vi "FPGA Main.vi"() -> ()   [LabVIEW 2013]
doc: "This FPGA Main VI contains a control loop running in parallel with an RT watchdog loop.\n- The Control Loop performs control calculations on four input channels in parallel, and outputs the results to four output channels.\n- The RT Watchdog Loop checks for a periodic 'pet' from the RT Main VI to ensure communications between RT and FPGA are maintained."
uses:
  controls/FPGA State.ctl
  controls/Control Configuration.ctl
  controls/Raw Values.ctl
  <vilib>/LabVIEW Targets/FPGA/cRIO/cRIO-9505/controls.llb/_nicrio_cRIO-9505_DriveStatus.ctl
  controls/Custom Controller Inputs.ctl
  controls/Controller Calcs.ctl
  controls/Observer Calcs.ctl
  controls/Other Calcs.ctl
  <vilib>/Platform/TimedLoop/XDataNode/timing_clust.ctl
  <vilib>/Platform/TimedLoop/XDataNode/nitl_modes.ctl
  <vilib>/Platform/TimedLoop/XDataNode/wakeup.ctl
  <vilib>/LabVIEW Targets/FPGA/cRIO/cRIO-9505/controls.llb/_nicrio_cRIO-9505_DriveDirection.ctl
  <vilib>/rvi/Emulation/niFpgaSctlEmulationGetInTimedLoop.vi
  <vilib>/rvi/Emulation/niFpgaEmulationReportErrorSimple.vi
  <vilib>/rvi/Emulation/niFpgaGetClockAttributes.vi
  <vilib>/rvi/Emulation/niFpgaCriticalErrorInLSC.vi
  <vilib>/rvi/Emulation/niFpgaProcessEmulError.vi
  <vilib>/rvi/eio/common/nirviEmuTemplateMethod_errors.vi
  <vilib>/rvi/eio/common/nirviEmuTemplatePropertyGet_noerrors.vi
  <vilib>/Platform/TimedLoop/XDataNode/XDataNode.xnode
  <vilib>/eio/EIONode/EIONode.xnode
  <vilib>/eio/EIOMethodNode/EIOMethodNode.xnode
  <vilib>/eio/EIOPropertyNode/EIOPropertyNode.xnode
  <vilib>/rvi/Analysis/measure/butterworth/XNode/niFpgaButterworthFilter.xnode
  <vilib>/Platform/TimedLoop/XDataNode/XDNodeRunTimeDep.lvlib
  <vilib>/rvi/eio/common/nirviEmuTemplatePropertyGet_errors.vi
  <vilib>/rvi/eio/common/nirviEmuTemplatePropertySet_errors.vi
  <vilib>/rvi/eio/common/nirviEmuTemplatePropertySet_noerrors.vi
panel:
  out "Other Calcs":T1
  out "Observer Calcs":T2
  out "Controller Calcs":T3
  in  "Reset Integrator":bool
  in  "Custom Controller Inputs":T4={"Other Controller Gains"={"kvc (N/m)"=3000.0, "ymod (-)"=0.0, "Mar (kg)"=0.0, "bp (kg/s)"=0.0, "Foff (N)"=0.0, "Fthresh (N)"=2.0}}
  in  "Mod1/AO4":fxp<+,16,3>
  in  "Trig AI":bool
  out "Vsup Present":bool
  out "Drive Fault":bool
  out "Drive Status":T5=enum."Disabled"
  out "Temp Fault":bool
  in  "Enable\nDrive":bool
  in  "Disable\nDrive":bool
  out "PWM Duty Cycle":i16
  out "F_Error (N)":fxp<+/-,40,11>
  in  "Force Sensor Gain (N/V)":fxp<+,20,6>=53.02703857421875
  in  "L12 Offset (mA)":fxp<+,18,4>=1.0
  in  "L12 Gain (mA/N)":fxp<+,16,2>=1.0
  out "Measured Force (N)":fxp<+,39,10>
  out "Controller\nOutput":fxp<+,18,3>
  in  "Channel 3 Setpoint":fxp<+/-,16,7>
  in  "Channel 2 Setpoint":fxp<+/-,20,7>
  in  "Channel 1 Setpoint  (Position)":fxp<+/-,20,7>=25.0
  in  "Channel 0 Setpoint (Force)":fxp<+/-,20,7>
  out "Watchdog Timed Out?":bool=TRUE
  in  "Enable Watchdog":bool
  in  "Pet Watchdog":bool
  in  "Watchdog Timeout Period (ticks)":u64=40000000 format="%.0p"
  out "Time Since Last Pet":u64
  in  "Manual Values":T6
  out "Output Values":T6
  out "Input Values":T6
  in  "Channel 3 Configuration":T7={"PID Gains"={"proportional gain (Kc)"=0.0, "integral gain (Kc*Ts/Ti)"=0.0, "derivative gain (Kc*Td/Ts)"=0.0}, "Output Range"={"output high"=10.0, "output low"=-10.0}}
  in  "Channel 2 Configuration":T7={"PID Gains"={"proportional gain (Kc)"=0.0, "integral gain (Kc*Ts/Ti)"=0.0, "derivative gain (Kc*Td/Ts)"=0.0}, "Output Range"={"output high"=10.0, "output low"=-10.0}}
  in  "Channel 1 Configuration":T7={"PID Gains"={"proportional gain (Kc)"=0.0, "integral gain (Kc*Ts/Ti)"=0.0, "derivative gain (Kc*Td/Ts)"=0.0}, "Output Range"={"output high"=10.0, "output low"=-10.0}}
  in  "Channel 0 Configuration":T7={"PID Gains"={"proportional gain (Kc)"=55.0, "integral gain (Kc*Ts/Ti)"=0.0, "derivative gain (Kc*Td/Ts)"=0.0}, "Output Range"={"output high"=50.0, "output low"=-50.0}}
  in  "New State":T8=enum."Control (PID)"
  out "Actual Loop Period (ticks)":u32
  out "Current FPGA State":T8=enum."Manual"
  in  "Change State":bool
  out "Input Error":bool
  out "Output Error":bool
  in  "Control Period (ticks)":u32
  # "General Settings"
  # "Manual Settings"
  # "Monitoring Values"
  # "Watchdog Settings"
  # "Control Settings"
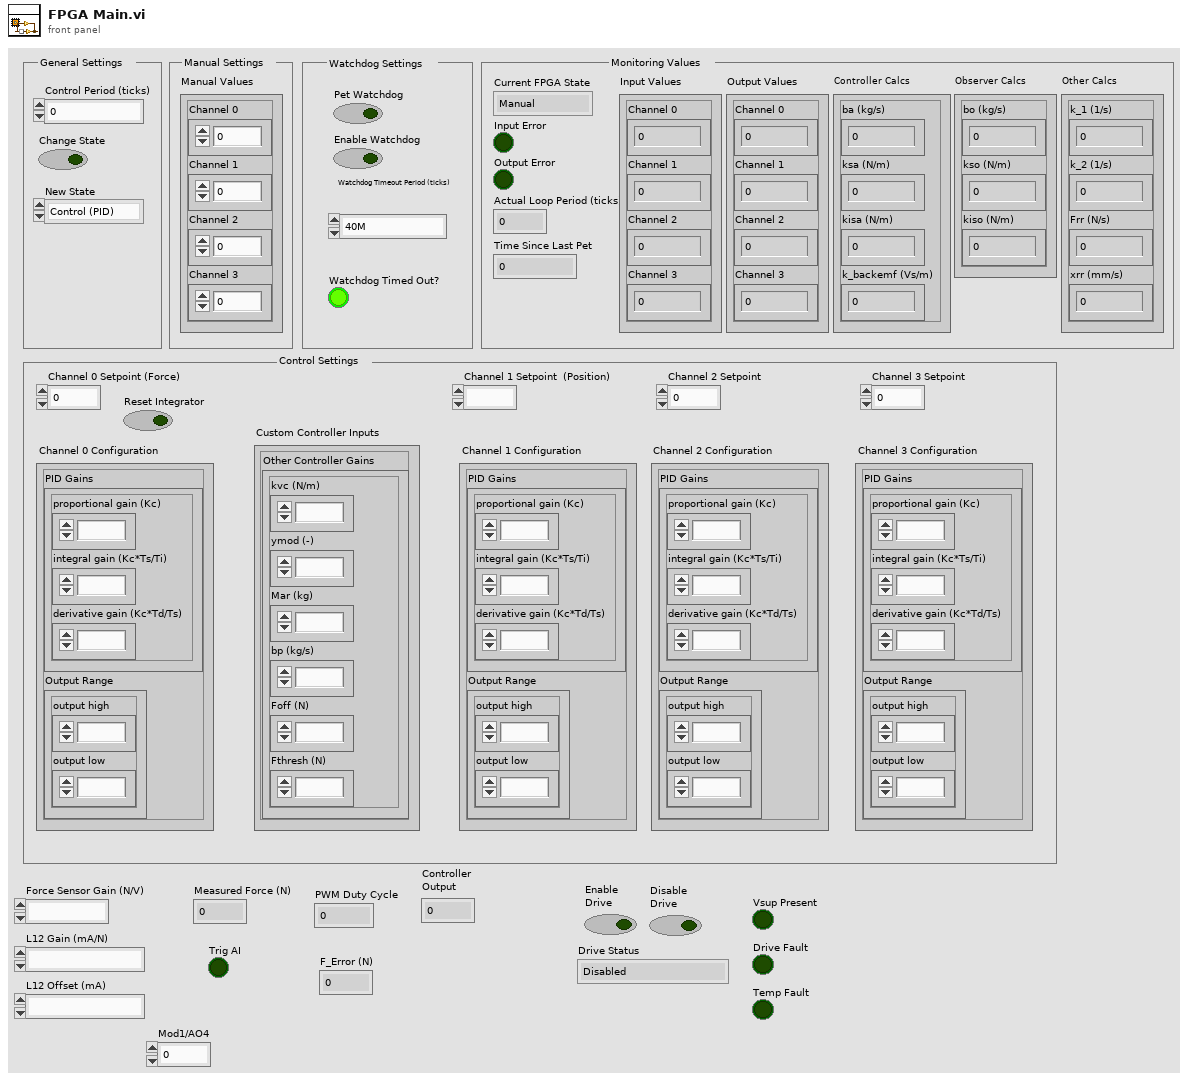
[diagram p1: front panel]
types:
  T1 = typedef "Other Calcs.ctl" = cluster{"k_1 (1/s)":fxp<+/-,20,7>, "k_2 (1/s)":fxp<+/-,20,7>, "Frr (N/s)":fxp<+/-,20,7>, "xrr (mm/s)":fxp<+/-,20,14>}
  T2 = typedef "Observer Calcs.ctl" = cluster{"bo (kg/s)":fxp<+/-,20,7>, "kso (N/m)":fxp<+/-,20,7>, "kiso (N/m)":fxp<+/-,20,7>}
  T3 = typedef "Controller Calcs.ctl" = cluster{"ba (kg/s)":fxp<+/-,20,7>, "ksa (N/m)":fxp<+/-,20,7>, "kisa (N/m)":fxp<+/-,20,7>, "k_backemf (Vs/m)":fxp<+/-,20,14>}
  T4 = typedef "Custom Controller Inputs.ctl" = cluster{"Other Controller Gains":cluster{"kvc (N/m)":fxp<+,16,12>, "ymod (-)":fxp<+/-,16,5>, "Mar (kg)":fxp<+/-,16,8>, "bp (kg/s)":fxp<+/-,16,5>, "Foff (N)":fxp<+/-,16,8>, "Fthresh (N)":fxp<+/-,16,5>}}
  T5 = typedef "_nicrio_cRIO-9505_DriveStatus.ctl" = enum8{"Enabled", "Disabled", "Disabled by Drive Fault", "Disabled by Temp. Fault", "Disabled by E-Stop", "Unknown"}
  T6 = typedef "Raw Values.ctl" = cluster{"Channel 0":fxp<+/-,20,7>, "Channel 1":fxp<+/-,20,7>, "Channel 2":fxp<+/-,20,7>, "Channel 3":fxp<+/-,20,14>}
  T7 = typedef "Control Configuration.ctl" = cluster{"PID Gains":cluster{"proportional gain (Kc)":fxp<+/-,16,8>, "integral gain (Kc*Ts/Ti)":fxp<+/-,16,8>, "derivative gain (Kc*Td/Ts)":fxp<+/-,16,8>}, "Output Range":cluster{"output high":fxp<+/-,16,7>, "output low":fxp<+/-,16,7>}}
  T8 = typedef "FPGA State.ctl" = enum16{"Safe State", "Manual", "Control (PID)"}
  T9 = typedef "XDNodeRunTimeDep.lvlib/timing_clust.ctl" = cluster{"Expected End [f-1]":u64, "Actual End [f-1]":u64, "Finished Late? [f-1]":bool, "Expected End [i-1]":u64, "Actual End [i-1]":u64, "Finished Late? [i-1]":bool, "Expected Start [i]":u64, "Actual Start [i]":u64, "Expected Start [f]":u64, "Actual Start [f]":u64, "Source Name":string, "Structure Name":string, "Period":i64, "Deadline":i64, "Offset":i64, "Start":i64, "Priority":i32, "Timeout":i32, "Mode":T10, "Wakeup Reason":T11, "Error":errorcluster, "Source Type":string, "Secondary Source Type":string, "Global End Time":u64, "Global Start Time":u64, "Frame Duration":u64, "Iteration Duration":u64, "Assigned CPU":i32, "I/O Scan Engine Mode":u32}
  T10 = typedef "XDNodeRunTimeDep.lvlib/nitl_modes.ctl" = enum32{"No Change", "Process missed periods, maintain original phase", "Discard missed periods, maintain original phase", "Process missed periods, ignore original phase", "Discard missed periods, ignore original phase"}
  T11 = typedef "XDNodeRunTimeDep.lvlib/wakeup.ctl" = enum32{"Normal", "Aborted", "Asynchronous wakeup", "Timing source error", "Timed loop error", "Timeout"}
  T12 = cluster{"kvc (N/m)":fxp<+,16,12>, "ymod (-)":fxp<+/-,16,5>, "Mar (kg)":fxp<+/-,16,8>, "bp (kg/s)":fxp<+/-,16,5>, "Foff (N)":fxp<+/-,16,8>, "Fthresh (N)":fxp<+/-,16,5>}
  T13 = cluster{fxp<+,1,1>, fxp<+,1,2>, fxp<+,2,2>, fxp<+,1,3>}
  T14 = typedef "_nicrio_cRIO-9505_DriveDirection.ctl" = enum8{"Clockwise", "Counterclockwise"}
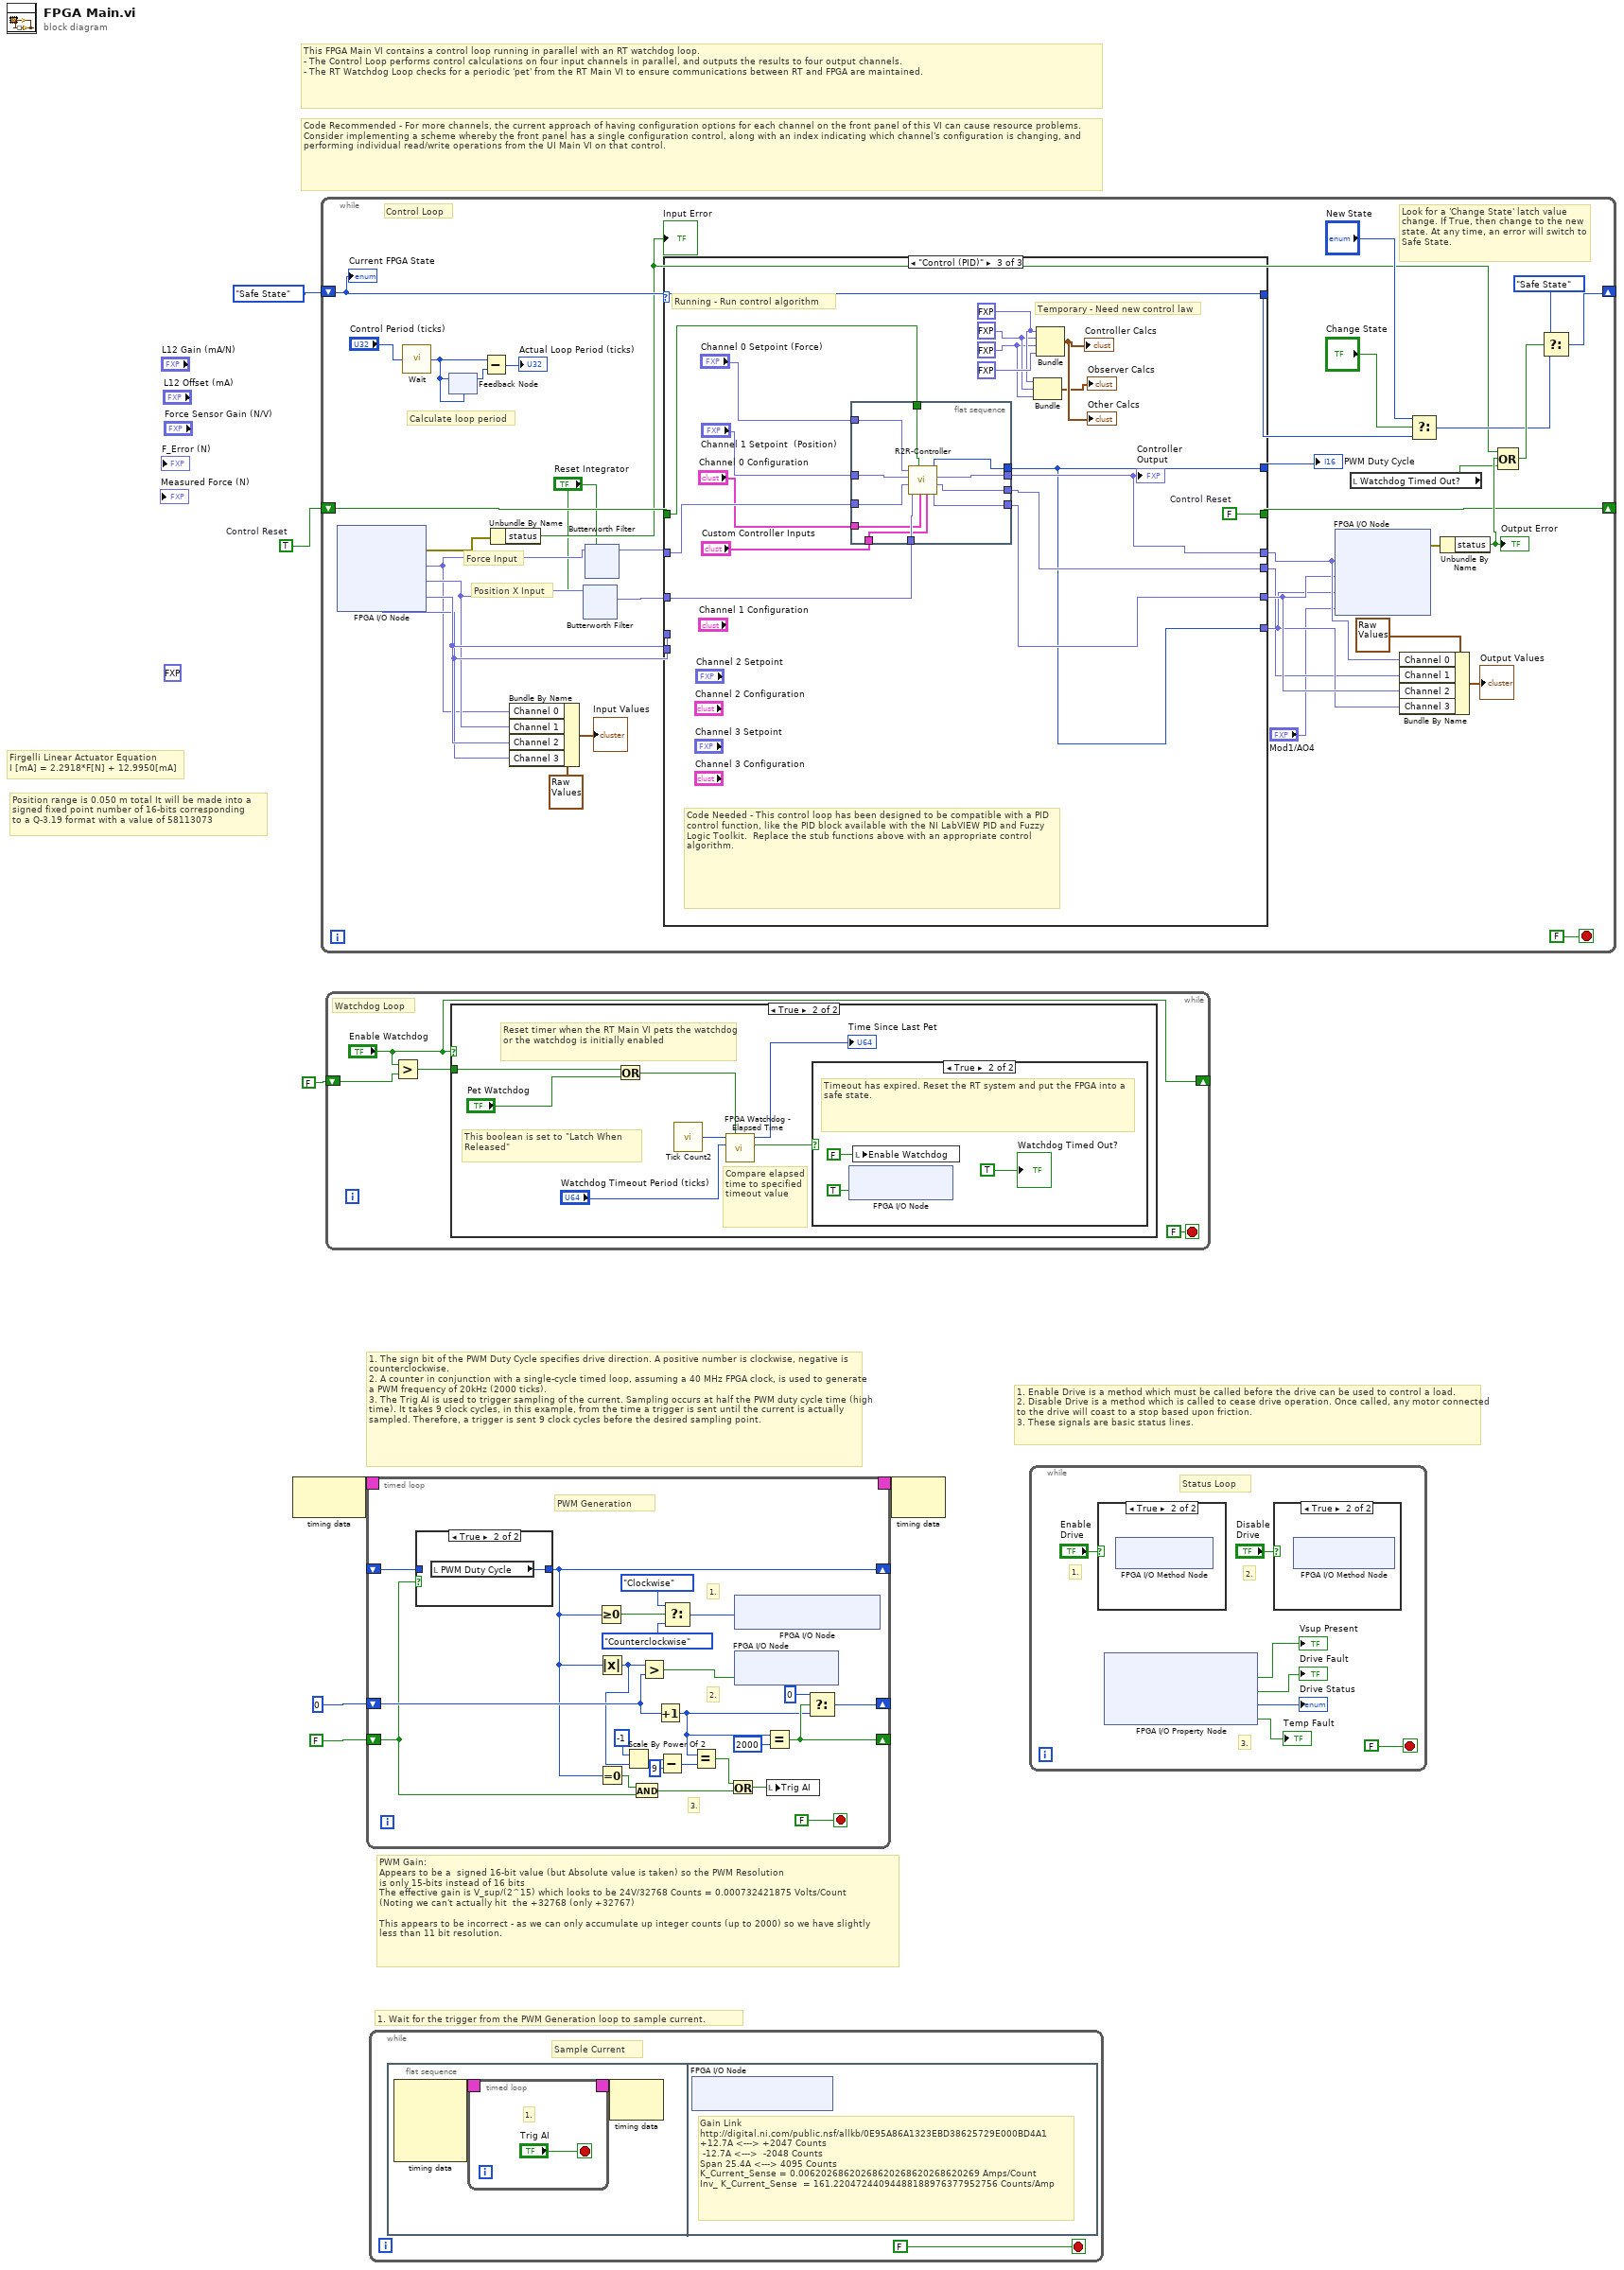
[diagram p0: block diagram]
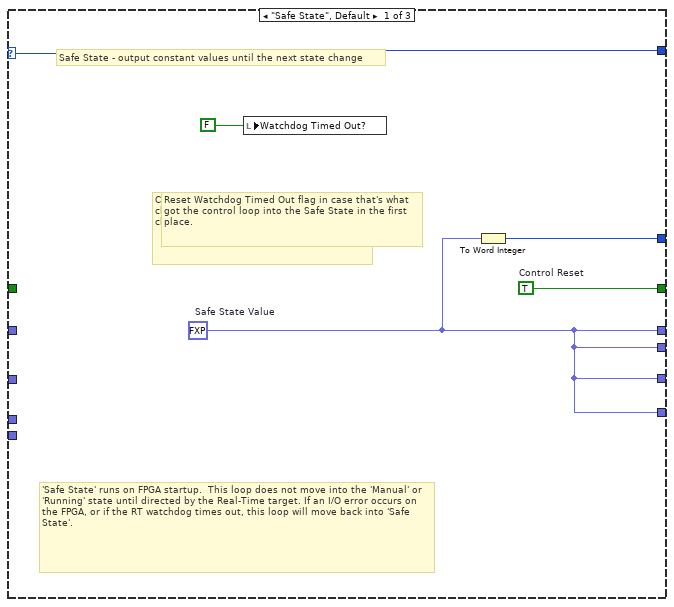
[diagram p7: hidden frame]
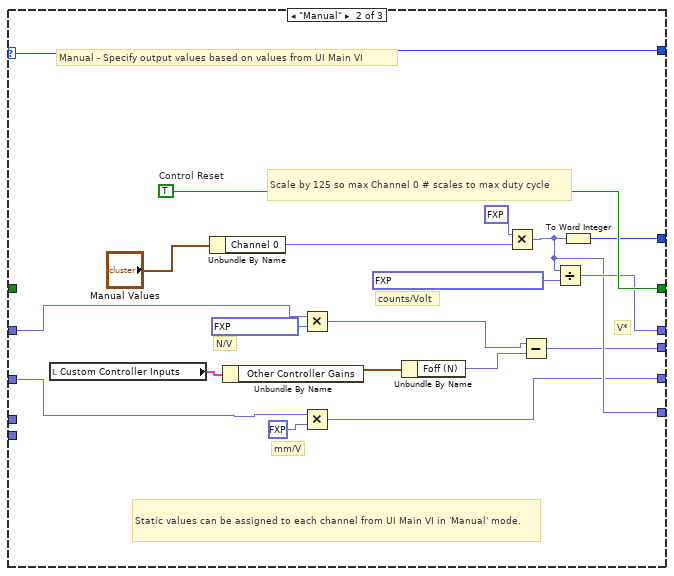
[diagram p8: hidden frame]
diagram:
  (unwired) fxp<+,18,3> 0.0 ("F (Raw Analog V)")
  w6 = TRUE  # Control Reset
  # "PWM Gain:\nAppears to be a  signed 16-bit value (but Absolute value is taken) so the PWM Resolution\nis only 15-bits instead of 16 bits\nThe effective gain is V_sup/(2^15) which looks to be 24V/32768 Counts = 0.000732421875 Volts/Count\n(Noting we can't actually hit  the +32768 (only +32767)\n\nThis appears to be incorrect - as we can only accumulate up integer counts (up to 2000) so we have slightly\nless than 11 bit resolution."
  # "1. Enable Drive is a method which must be called before the drive can be used to control a load.\n2. Disable Drive is a method which is called to cease drive operation. Once called, any motor connected to the drive will coast to a stop based upon friction.\n3. These signals are basic status lines."
  # "1. Wait for the trigger from the PWM Generation loop to sample current."
  # "1. The sign bit of the PWM Duty Cycle specifies drive direction. A positive number is clockwise, negative is counterclockwise.\n2. A counter in conjunction with a single-cycle timed loop, assuming a 40 MHz FPGA clock, is used to generate a PWM frequency of 20kHz (2000 ticks).\n3. The Trig AI is used to trigger sampling of the current. Sampling occurs at half the PWM duty cycle time (high time). It takes 9 clock cycles, in this example, from the time a trigger is sent until the current is actually sampled. Therefore, a trigger is sent 9 clock cycles before the desired sampling point."
  # "Position range is 0.050 m total It will be made into a \nsigned fixed point number of 16-bits corresponding \nto a Q-3.19 format with a value of 58113073"
  # "Firgelli Linear Actuator Equation\nI [mA] = 2.2918*F[N] + 12.9950[mA]"
  # "Code Recommended - For more channels, the current approach of having configuration options for each channel on the front panel of this VI can cause resource problems.  Consider implementing a scheme whereby the front panel has a single configuration control, along with an index indicating which channel's configuration is changing, and performing individual read/write operations from the UI Main VI on that control."
  # "This FPGA Main VI contains a control loop running in parallel with an RT watchdog loop.\n- The Control Loop performs control calculations on four input channels in parallel, and outputs the results to four output channels.\n- The RT Watchdog Loop checks for a periodic 'pet' from the RT Main VI to ensure communications between RT and FPGA are maintained."
  n1 = node-c288() -> (w4:T9)  [unwired: 1 out]
  n2 = while {
    shift-right: [w39] -> _
    shift-left: FPGA_State."Safe State" ("FPGA State") -> [w30]
    shift-right: [w36] -> _
    shift-left: w6 -> [w35]
    stop <- FALSE stop-if-true
    # "Position X Input"
    # "Force Input"
    # "Calculate loop period"
    # "Look for a 'Change State' latch value change. If True, then change to the new state. At any time, an error will switch to Safe State."
    # "Control Loop"
    n3 = xnode "FPGA I/O Node"() -> ("error out"=w43:errorcluster, "Mod1/AI0"=w10:fxp<+,18,3>, "Mod1/AI1"=w12:fxp<+,18,3>, "Mod1/AI2"=w28:fxp<+,18,3>, "Mod1/AI3"=w27:fxp<+,18,3>)  [unwired: 5 in, 4 out]
    n4 = call "Wait"("Count(Ticks)"="Control Period (ticks)") -> ("Tick Count(Ticks)"=w20:u32)
    n5 = feedback-in #1(w20) -> ()
    n6 = feedback #1(w20) -> (w19:u32)
    n7 = Subtract(x=w20, y=w19) -> (x-y=→"Actual Loop Period (ticks)":u32)
    n8 = Unbundle By Name(w43) -> ("status"=w29:bool)
    "Input Error" <- w29
    n9 = Bundle By Name(cluster=T6 {"Channel 0"=0.0, "Channel 1"=0.0, "Channel 2"=0.0, "Channel 3"=0.0} ("Raw Values"), "Channel 0"=w10, "Channel 1"=w12, "Channel 2"=w28, "Channel 3"=w27) -> (→"Input Values":T6)
    n10 = xnode "Butterworth Filter"("input data"=w12, "reset"="Reset Integrator") -> ("output data"=w11:fxp<+/-,23,8>)  [unwired: 1 in]
    n11 = xnode "Butterworth Filter"("input data"=w10, "reset"="Reset Integrator") -> ("output data"=w9:fxp<+/-,23,8>)  [unwired: 1 in]
    n12 = case shown="\"Control (PID)\"" w30 {
      selector: w30 -> [w64 w83 w102]
      tunnel: w9 -> [_ w74 w99]
      tunnel: [w61 w77 w94] -> w26
      tunnel: [w64 w83 w102] -> w34
      tunnel: [w65 w84 w103] -> w36
      tunnel: w35 -> [_ _ w101]
      tunnel: w11 -> [_ w72 w96]
      tunnel: w28 -> [_ _ _]
      tunnel: w27 -> [_ _ _]
      tunnel: [w61 w66 w93] -> w15
      tunnel: [w61 w71 w92] -> w25
      tunnel: [w61 w76 w91] -> w24
      tunnel: [w62 w81 w91] -> w14
      frame "Safe State", Default {
        w61 = fxp<+/-,20,7> 0.0  # Safe State Value
        w65 = TRUE  # Control Reset
        # "'Safe State' runs on FPGA startup.  This loop does not move into the 'Manual' or 'Running' state until directed by the Real-Time target. If an I/O error occurs on the FPGA, or if the RT watchdog times out, this loop will move back into 'Safe State'."
        # "Reset Watchdog Timed Out flag in case that's what got the control loop into the Safe State in the first place."
        # "Safe State - output constant values until the next state change"
        # "Code Recommended - Modify this code to change the safe state value for each channel."
        n13 = local write "Watchdog Timed Out?"(FALSE ("Watchdog Timed Out?")) -> ()
        n14 = To Word Integer(number=w61) -> (16bit integer=w62:i16)
      }
      frame "Manual" {
        w84 = TRUE  # Control Reset
        # "N/V"
        # "mm/V"
        # "V*"
        # "counts/Volt"
        # "Scale by 125 so max Channel 0 # scales to max duty cycle"
        # "Manual - Specify output values based on values from UI Main VI"
        # "Static values can be assigned to each channel from UI Main VI in 'Manual' mode."
        n15 = local read "Custom Controller Inputs"() -> (w70:T4)
        n16 = Unbundle By Name("Manual Values") -> ("Channel 0"=w79:fxp<+/-,20,7>)
        n17 = Unbundle By Name(w70) -> ("Other Controller Gains"=w69:T12)
        n18 = Multiply(x=w74, y=fxp<+,20,6> 53.02685546875) -> (x*y=w68:fxp<+/-,43,14>)
        n19 = Multiply(x=w72, y=fxp<+,12,4> 10.0) -> (x*y=w71:fxp<+/-,35,12>)
        n20 = Unbundle By Name(w69) -> ("Foff (N)"=w67:fxp<+/-,16,8>)
        n21 = Multiply(x=fxp<+/-,20,8> 125.0, y=w79) -> (x*y=w76:fxp<+/-,40,15>)
        n22 = Subtract(x=w68, y=w67) -> (x-y=w66:fxp<+/-,44,15>)
        n23 = Divide(x=w76, y=fxp<+/-,40,15> 83.33199998736382) -> (x/y=w77:fxp<+/-,64,40>)
        n24 = To Word Integer(number=w76) -> (16bit integer=w81:i16)
      }
      frame "Control (PID)" {
        w86 = fxp<+,2,2> 3.0
        w88 = fxp<+,1,1> 1.0
        w87 = fxp<+,1,2> 2.0
        w103 = FALSE  # Control Reset
        # "Temporary - Need new control law"
        # "Running - Run control algorithm"
        # "Code Needed - This control loop has been designed to be compatible with a PID control function, like the PID block available with the NI LabVIEW PID and Fuzzy Logic Toolkit.  Replace the stub functions above with an appropriate control algorithm."
        n25 = flat-sequence {
          tunnel: "Channel 0 Setpoint (Force)" -> [w113]
          tunnel: w101 -> [w114]
          tunnel: w99 -> [w111]
          tunnel: [w106] -> w94
          tunnel: "Channel 0 Configuration" -> [w109]
          tunnel: "Custom Controller Inputs" -> [w108]
          tunnel: "Channel 1 Setpoint  (Position)" -> [w112]
          tunnel: w96 -> [w110]
          tunnel: [w107] -> w91
          tunnel: [w105] -> w93
          tunnel: [w104] -> w92
          frame #0 {
            n26 = call "R2R-Controller.vi"("Custom Controller Inputs"=w108, "Gain Configuration"=w109, "Reset Integrator"=w114, "X (Raw Analog V)"=w110, "F (Raw Analog V)"=w111, "X* (mm)"=w112, "F* (N)"=w113) -> ("Xmeas (mm)"=w104:fxp<+,30,7>, "Fmeas (N)"=w105:fxp<+/-,40,11>, "V*(V)"=w106:fxp<+/-,53,13>, "PWM Duty Cycle"=w107:i16)  [unwired: 1 out]
          }
        }
        n27 = Bundle(w88, w87, w86) -> (→"Observer Calcs":cluster{fxp<+,1,1>, fxp<+,1,2>, fxp<+,2,2>})  [unwired: 1 in]
        n28 = Bundle(w88, w87, w86, fxp<+,1,3> 4.0) -> (→"Controller Calcs" →"Other Calcs":T13)  [unwired: 1 in]
        "Controller\nOutput" <- w94
      }
    }
    "PWM Duty Cycle" <- w14
    n29 = xnode "FPGA I/O Node"("Mod1/AO0"=w26, "Mod1/AO2"=w25, "Mod1/AO3"=w24, "Mod1/AO4"="Mod1/AO4") -> ("error out"=w42:errorcluster)  [unwired: 5 in, 4 out]
    n30 = local read "Watchdog Timed Out?"() -> (w21:bool)
    n31 = Bundle By Name(cluster=T6 {"Channel 0"=0.0, "Channel 1"=0.0, "Channel 2"=0.0, "Channel 3"=0.0} ("Raw Values"), "Channel 0"=w26, "Channel 1"=w15, "Channel 2"=w25, "Channel 3"=w24) -> (→"Output Values":T6)
    n32 = Select(t="New State", s="Change State", f=w34) -> (s? t:f=w31:T8)
    n33 = Unbundle By Name(w42) -> ("status"=w41:bool)
    "Output Error" <- w41
    n34 = Compound Arithmetic op=OR(w29, w41, w21) -> (w38:bool)
    n35 = Select(t=FPGA_State."Safe State" ("FPGA State"), s=w38, f=w31) -> (s? t:f=w39:T8)
    "Current FPGA State" <- w30
  }
  n36 = while "RT Watchdog Loop" {
    shift-right: ["Enable Watchdog"] -> _
    shift-left: FALSE ("Enable RT Watchdog") -> [w118]
    stop <- FALSE stop-if-true
    # "Watchdog Loop"
    n37 = Greater?(x="Enable Watchdog", y=w118) -> (0:w115:bool)
    n38 = case shown="True" "Enable Watchdog" {
      tunnel: w115 -> [_ w121]
      frame False {
        # "This loop has to be explicitly enabled from the RT Main VI.  This reduces the possiblity of an endless reboot cycle."
      }
      frame True {
        # "This boolean is set to \"Latch When Released\""
        # "Compare elapsed time to specified timeout value"
        # "Reset timer when the RT Main VI pets the watchdog or the watchdog is initially enabled"
        n39 = Or(x=w121, y="Pet Watchdog") -> (x .or. y?=w120:bool)
        n40 = call "Tick Count2"() -> ("Tick Count(Ticks)"=w124:u32)
        n41 = call "FPGA Watchdog - Elapsed Time.vi"("Reset"=w120, "Timeout Period"="Watchdog Timeout Period (ticks)", "Current Time"=w124) -> ("Timeout"=w119:bool, "Elapsed Time"=→"Time Since Last Pet":u64)  [unwired: 7 in]
        n42 = case shown="True" w119 {
          frame False {
            # "Timeout has not expired."
          }
          frame True {
            # "Timeout has expired. Reset the RT system and put the FPGA into a safe state."
            n43 = xnode "FPGA I/O Node"("System Reset"=TRUE ("RT Reset on Watchdog Failure?")) -> ()  [unwired: 1 in, 1 out]
            n44 = local write "Enable Watchdog"(FALSE ("Enable RT Watchdog")) -> ()
            "Watchdog Timed Out?" <- TRUE ("Watchdog Timed Out?")
          }
        }
      }
    }
  }
  n45 = timed-loop {
    timing: w4 -> [_]
    timing-out: [_] -> w3
    shift-right: [w149] -> _
    shift-left: i16 0 -> [w152]
    shift-right: [w148] -> _
    shift-left: FALSE -> [w145]
    shift-right: [w129] -> _
    shift-left: _ -> [w147]
    stop <- FALSE stop-if-true
    # "3."
    # "2."
    # "1."
    # "PWM Generation"
    n46 = case shown="True" w145 {
      tunnel: [w153 w154] -> w129
      tunnel: w147 -> [w153 _]
      frame False {
      }
      frame True {
        n47 = local read "PWM Duty Cycle"() -> (w154:i16)
      }
    }
    n48 = Greater Or Equal To 0?(x=w129) -> (x >= 0?=w141:bool)
    n49 = Absolute Value(x=w129) -> (abs(x)=w131:i16)
    n50 = Equal To 0?(x=w129) -> (x = 0?=w146:bool)
    n51 = Scale By Power Of 2(n=i8 -1, x=w131) -> (x*2^n=w134:i16)
    n52 = And(x=w146, y=w145) -> (x .and. y?=w142:bool)
    n53 = Greater?(x=w131, y=w152) -> (0:w138:bool)
    n54 = Increment(x=w152) -> (x+1=w144:i16)
    n55 = Subtract(x=w134, y=i8 9) -> (x-y=w133:i16)
    n56 = Select(t=_nicrio_cRIO-9505_DriveDirection."Clockwise" ("Drive Direction"), s=w141, f=_nicrio_cRIO-9505_DriveDirection."Counterclockwise" ("Drive Direction")) -> (s? t:f=w137:T14)
    n57 = Equal?(x=w144, y=w133) -> (x = y?=w143:bool)
    n58 = Or(x=w143, y=w142) -> (x .or. y?=w136:bool)
    n59 = xnode "FPGA I/O Node"("Mod2/Drive Direction"=w137) -> ()  [unwired: 1 in, 1 out]
    n60 = xnode "FPGA I/O Node"("Mod2/Motor"=w138) -> ()  [unwired: 1 in, 1 out]
    n61 = Equal?(x=w144, y=i16 2000) -> (x = y?=w148:bool)
    n62 = local write "Trig AI"(w136) -> ()
    n63 = Select(t=i16 0, s=w148, f=w144) -> (s? t:f=w149:i16)
  }
  n64 = while {
    stop <- FALSE stop-if-true
    # "Sample Current"
    n65 = flat-sequence {
      frame #0 {
        n66 = node-c288() -> (w159:T9)  [unwired: 4 out]
        n67 = timed-loop {
          timing: w159 -> [_]
          timing-out: [_] -> w158
          stop <- "Trig AI" stop-if-true
          # "1."
        }
        n68 = node-c288(w158) -> ()  [unwired: 1 out]
      }
      frame #1 {
        # "Gain Link\nhttp://digital.ni.com/public.nsf/allkb/0E95A86A1323EBD38625729E000BD4A1\n+12.7A <---> +2047 Counts\n -12.7A <--->  -2048 Counts\nSpan 25.4A <---> 4095 Counts\nK_Current_Sense = 0.00620268620268620268620268620269 Amps/Count\nInv_ K_Current_Sense  = 161.22047244094488188976377952756 Counts/Amp"
        n69 = xnode "FPGA I/O Node"() -> ()  [unwired: 1 in, 2 out]
      }
    }
  }
  n70 = node-c288(w3) -> ()  [unwired: 1 out]
  n71 = while {
    stop <- FALSE stop-if-true
    # "3."
    # "2."
    # "1."
    # "Status Loop"
    n72 = case shown="True" "Enable\nDrive" {
      frame False {
      }
      frame True {
        n73 = xnode "FPGA I/O Method Node"() -> ()  [unwired: 1 in, 1 out]
      }
    }
    n74 = xnode "FPGA I/O Property Node"() -> ("Vsup Present"=→"Vsup Present":bool, "Drive Fault"=→"Drive Fault":bool, "Drive Status"=→"Drive Status":T5, "Over Temperature Fault"=→"Temp Fault":bool)  [unwired: 1 in, 1 out]
    n75 = case shown="True" "Disable\nDrive" {
      frame False {
      }
      frame True {
        n76 = xnode "FPGA I/O Method Node"() -> ()  [unwired: 1 in, 1 out]
      }
    }
  }
